vi "Animated GIF Reader Example.vi"() -> ()   [LabVIEW 2020]
panel:
  in  "stop":bool
  out "Picture":picture
  in  "path to GIF file":path
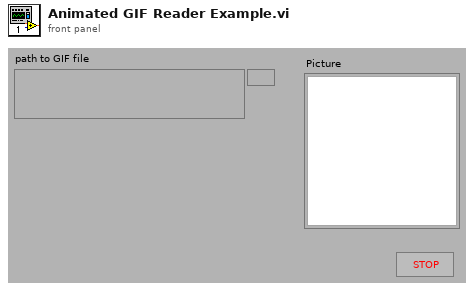
[diagram p1: front panel]
types:
  T1 = typedef "imagedata.ctl" = cluster{"image type":i32, "image depth":i32, "image":u8[], "mask":u8[], "colors":u32[], "Rectangle":cluster{"left":i16, "top":i16, "right":i16, "bottom":i16}}
  T2 = cluster{"left":i16, "top":i16, "right":i16, "bottom":i16}
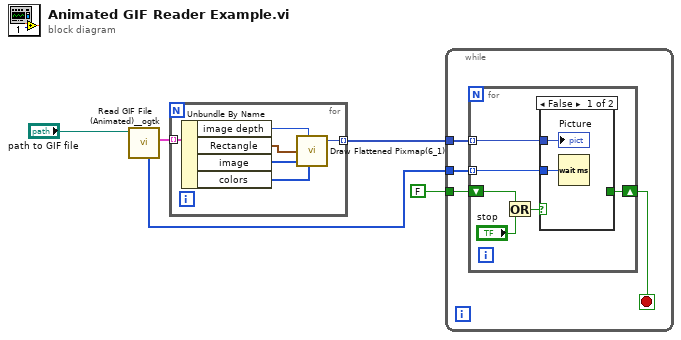
[diagram p0: block diagram]
diagram:
  n1 = call <userlib>:"Read GIF File (Animated)__ogtk.vi"("path to GIF file"="path to GIF file") -> ("images data"=w4:T1[], "Delay (ms)"=w2:u32[])  [unwired: 6 in, 3 out]
  n2 = for {
    tunnel: w4 -> [w11] mode=indexing
    tunnel: [w6] -> w3 mode=indexing
    n3 = Unbundle By Name(w11) -> ("image depth"=w7:i32, "Rectangle"=w10:T2, "image"=w9:u8[], "colors"=w8:u32[])
    n4 = call <vilib>:"Draw Flattened Pixmap(6_1).vi"("bit depth(8)"=w7, "rect"=w10, "flattened pixmap data"=w9, "color table"=w8) -> ("new picture"=w6:picture)  [unwired: 5 in]
  }
  n5 = while {
    tunnel: w3 -> [w15]
    tunnel: w2 -> [w14]
    tunnel: FALSE -> [w12]
    stop <- w13 stop-if-true
    n6 = for {
      tunnel: w15 -> [w21] mode=indexing
      tunnel: w14 -> [w20] mode=indexing
      shift-right: [w16] -> w13
      shift-left: w12 -> [w17]
      n7 = Or(x=w17, y="stop") -> (x .or. y?=w18:bool)
      n8 = case shown="False" w18 {
        selector: w18 -> [_ w24]
        tunnel: w21 -> [w23 _]
        tunnel: w20 -> [w22 _]
        tunnel: [_ w24] -> w16
        frame False {
          n9 = Wait (ms)(milliseconds to wait=w22) -> ()  [unwired: 1 out]
          "Picture" <- w23
        }
        frame True {
        }
      }
    }
  }
